vi "tp4-2.vi"() -> ()   [LabVIEW 2013]
uses:
  <vilib>/sound2/lvsound2.llb/Sound Input Read (DBL).vi
panel:
  out "Numeric":dbl
  in  "Frecuencia":dbl=150.0
  out "Boolean":bool
  in  "stop":bool
  out "Waveform Graph":dbl[](graph)
  in  "Cluster":T1={"Sample rate S/s"=44100.0, "Number of channels"=1.0, "bits per sample"=16.0}
  in  "Buffer de lectura":dbl=11025.0
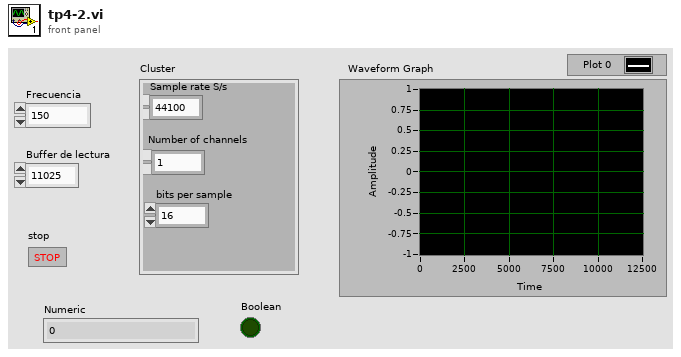
[diagram p1: front panel]
types:
  T1 = cluster{"Sample rate S/s":dbl, "Number of channels":dbl, "bits per sample":dbl}
  T2 = typedef "Sound Input Task ID.ctl" = u32
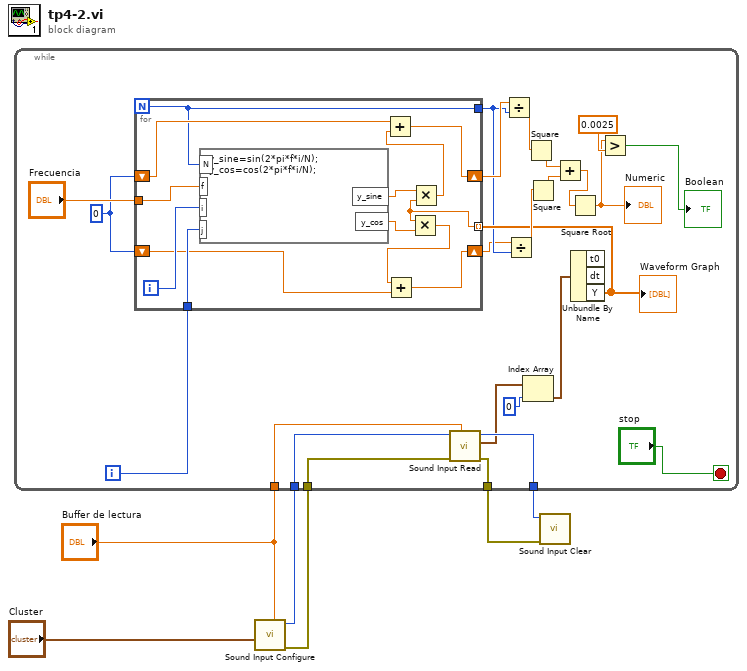
[diagram p0: block diagram]
diagram:
  n1 = call <vilib>:"Sound Input Configure.vi"("number of samples/ch"="Buffer de lectura", "sound format"="Cluster") -> ("error out"=w5:errorcluster, "task ID"=w4:T2)  [unwired: 8 in]
  n2 = while {
    tunnel: [w30] -> w6
    tunnel: w5 -> [w29]
    tunnel: w4 -> [w28]
    tunnel: [w27] -> w3
    tunnel: "Buffer de lectura" -> [w26]
    i -> [w21]
    stop <- "stop" stop-if-true
    w19 = 0
    n3 = call-poly <vilib>:"Sound Input Read.vi"("number of samples/ch"=w26, "error in (no error)"=w29, "task ID"=w28) -> ("error out"=w30:errorcluster, "data"=w25:waveform(dbl)[], "task ID out"=w27:T2)  [unwired: 6 in]
    n4 = Index Array(array=w25, index=0) -> (element=w23:waveform(dbl))
    n5 = Unbundle By Name(w23) -> ("Y"=w14:dbl[])  [unwired: 2 out]
    "Waveform Graph" <- w14
    n6 = for {
      N -> [w31]
      tunnel: w21 -> [w42]
      tunnel: w14 -> [w39] mode=indexing
      shift-right: [w32] -> w11
      shift-right: [w33] -> w9
      shift-left: w19 -> [w36]
      shift-left: w19 -> [w35]
      tunnel: "Frecuencia" -> [w38]
      tunnel: [w31] -> w10
      i -> [w43]
      n7 = formula code="y_sine=sin(2*pi*f*i/N);\ny_cos=cos(2*pi*f*i/N);"("i"=w43, "j"=w42, "N"=w31, "f"=w38) -> ("y_sine"=w41:dbl, "y_cos"=w40:dbl)
      n8 = Multiply(x=w39, y=w40) -> (x*y=w37:dbl)
      n9 = Add(x=w37, y=w36) -> (x+y=w33:dbl)
      n10 = Multiply(x=w41, y=w39) -> (x*y=w34:dbl)
      n11 = Add(x=w35, y=w34) -> (x+y=w32:dbl)
    }
    n12 = Divide(x=w11, y=w10) -> (x/y=w18:dbl)
    n13 = Divide(x=w9, y=w10) -> (x/y=w17:dbl)
    n14 = Square(x=w18) -> (x^2=w16:dbl)
    n15 = Square(x=w17) -> (x^2=w15:dbl)
    n16 = Add(x=w16, y=w15) -> (x+y=w8:dbl)
    n17 = Square Root(x=w8) -> (sqrt(x)=w12:dbl)
    "Numeric" <- w12
    n18 = Greater?(x=w12, y=0.0025) -> (0:→"Boolean":bool)
  }
  n19 = call <vilib>:"Sound Input Clear.vi"("error in (no error)"=w6, "task ID"=w3) -> ()  [unwired: 9 in, 1 out]
